vi "CurrentCalculation.vi"(8 "ReadBackCurrent":dbl, 9 "iter":i32, 10 "daguas max current":dbl, 11 "PolarityStatus":bool) -> (1 "PositiveBool":bool, 2 "SameSignBool":bool, 3 "Setcurrent":dbl)   [LabVIEW 2013]
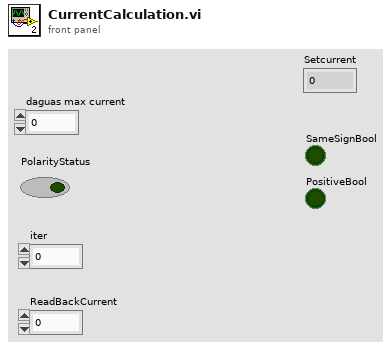
[diagram p1: front panel]
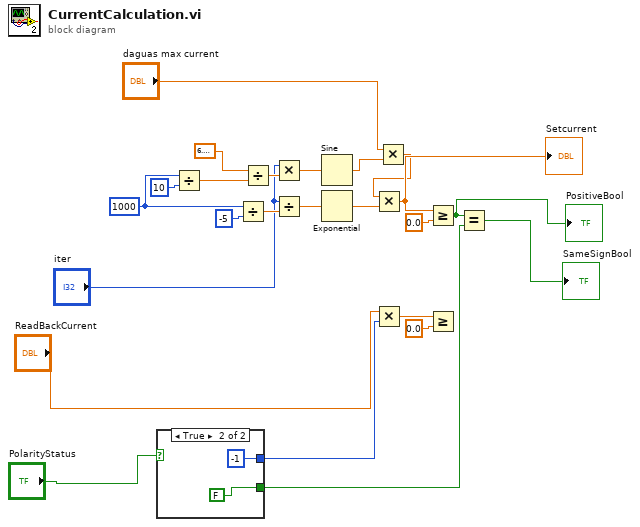
[diagram p0: block diagram]
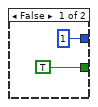
[diagram p2: hidden frame]
diagram:
  w13 = 1000
  n1 = case shown="True" "PolarityStatus" {
    tunnel: [1 -1] -> w12
    tunnel: [TRUE FALSE] -> w1
    frame False {
    }
    frame True {
    }
  }
  n2 = Divide(x=w13, y=10) -> (x/y=w17:dbl)
  n3 = Divide(x=w13, y=-5) -> (x/y=w19:dbl)
  n4 = Divide(x=6.283185307179586, y=w17) -> (x/y=w24:dbl)
  n5 = Multiply(x="iter", y=w24) -> (x*y=w23:dbl)
  n6 = Divide(x="iter", y=w19) -> (x/y=w22:dbl)
  n7 = Sine(x=w23) -> (sin(x)=w10:dbl)
  n8 = Exponential(1:w22) -> (0:w21:dbl)
  n9 = Multiply(x="ReadBackCurrent", y=w12) -> (x*y=w11:dbl)
  n10 = Multiply(x="daguas max current", y=w10) -> (x*y=w9:dbl)
  n11 = Multiply(x=w9, y=w21) -> (x*y=w14:dbl)
  "Setcurrent" <- w14
  n12 = Greater Or Equal?(x=w14, y=0.0) -> (x >= y?=w2:bool)
  "PositiveBool" <- w2
  n13 = Greater Or Equal?(x=w11, y=0.0) -> ()  [unwired: 1 out]
  n14 = Equal?(x=w2, y=w1) -> (x = y?=→"SameSignBool":bool)
